vi "Write Last Controlword.vi"(8 "error in (no error)":errorcluster, 10 "Controlword":string(combo), 11 "Motor Base in":refnum<class "Motor Base.lvclass">) -> (0 "error out":errorcluster, 3 "Motor Base out":refnum<class "Motor Base.lvclass">)   [LabVIEW 2016, in "Motor Base.lvlib" / "Motor Base.lvclass"]
uses:
  Motor Base.lvclass
  Motor Base.lvclass/Motor Base.ctl
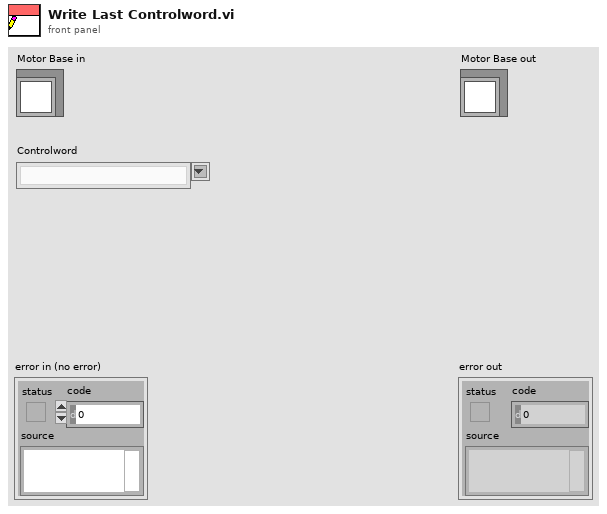
[diagram p1: front panel]
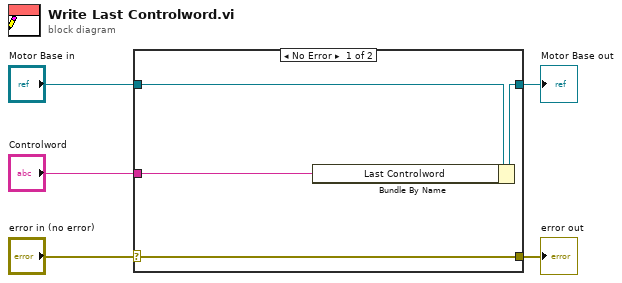
[diagram p0: block diagram]
diagram:
  n1 = case shown="No Error" "error in (no error)" {
    selector: "error in (no error)" -> [w9 w10]
    tunnel: [w9 w10] -> w4
    tunnel: [w7 w11] -> w2
    tunnel: "Motor Base in" -> [w8 w11]
    tunnel: "Controlword" -> [w6 _]
    frame No Error {
      n2 = Bundle By Name(cluster=w8, "Last Controlword"=w6) -> (w7:refnum<class "Motor Base.lvclass">)
    }
    frame Error {
    }
  }
  "error out" <- w4
  "Motor Base out" <- w2
